vi "Version_4.9_8_on-chip_valves_for25ulSyringe_withModfied_Plunging.vi"() -> ()   [LabVIEW 2020] (continued)
                                n5545 = local read "VISA Refnum in\nfor Pump"() -> (w5935:refnum<visa-resource-name>)
                                n5546 = local read "Volume of Syringe"() -> (w5932:dbl)
                                n5547 = call "GoToAbsolutePosition(SubVI).vi"("Absolute Volume Position in Syringe (in ul)"=0.0, "Volume of Syringe"=w5932, "Resolution of Pumping"=T2."Standard Pumping", "Flow Rate (ul/min)"=150.0, "VISA Refnum in"=w5935) -> ()  [unwired: 6 in, 1 out]
                                }
                                frame #7 {
                                n5548 = local read "Stopper that ends \nthe main loops"() -> (w5936:bool)
                                n5549 = local read "VISA Refnum in\nfor Pump"() -> (w5937:refnum<visa-resource-name>)
                                n5550 = case shown="True" w5936 {
                                frame False {
                                }
                                frame True {
                                n5551 = local read "VISA Refnum in\nfor Pump"() -> (w5938:refnum<visa-resource-name>)
                                n5552 = call "HardStopCurrentProcess (SubVI).vi"("VISA Refnum in"=w5938) -> ()  [unwired: 11 in]
                                }
                                }
                                n5553 = call "ProcessCompletionWaiter (SubVI).vi"("VISA Refnum in"=w5937) -> ()  [unwired: 11 in]
                                }
                                }
                                }
                              }
                            }
                          }
                          frame #21 {
                            n5554 = local read "VISA Refnum in\nfor Pump"() -> (w5940:refnum<visa-resource-name>)
                            n5555 = local read "Port for \nC2-Elution"() -> (w5939:string)
                            n5556 = call "PortChanger (SubVI).vi"("Port Number"=w5939, "VISA Refnum in"=w5940) -> ()  [unwired: 10 in]
                          }
                          frame #22 {
                            n5557 = local read "VISA Refnum in\nfor Pump"() -> (w5941:refnum<visa-resource-name>)
                            n5558 = call "ProcessCompletionWaiter (SubVI).vi"("VISA Refnum in"=w5941) -> ()  [unwired: 11 in]
                          }
                          frame #23 {
                            n5559 = local read "Buffer-C2 PickUp \nFlow Rate (ul/min)"() -> (w5945:dbl)
                            n5560 = local read "Buffer-C2 Pumping\nResolution"() -> (w5944:T2)
                            n5561 = local read "VISA Refnum in\nfor Pump"() -> (w5947:refnum<visa-resource-name>)
                            n5562 = local read "Buffer-C2 Volume \nto be Pumped"() -> (w5943:dbl)
                            n5563 = local read "Volume of Syringe"() -> (w5946:dbl)
                            n5564 = call "RPickUp(SubVI).vi"("Volume to be picked up"=w5943, "Volume of Syringe"=w5946, "Resolution of PickUP"=w5944, "PickUp Flow Rate (ul/min)"=w5945, "VISA Refnum in"=w5947) -> ()  [unwired: 6 in, 1 out]
                            n5565 = local write "SEC On"(TRUE ("SEC On")) -> ()
                          }
                          frame #24 {
                            n5566 = local read "Stopper that ends \nthe main loops"() -> (w5948:bool)
                            n5567 = local read "VISA Refnum in\nfor Pump"() -> (w5949:refnum<visa-resource-name>)
                            n5568 = case shown="True" w5948 {
                              frame False {
                              }
                              frame True {
                                n5569 = local read "VISA Refnum in\nfor Pump"() -> (w5950:refnum<visa-resource-name>)
                                n5570 = call "HardStopCurrentProcess (SubVI).vi"("VISA Refnum in"=w5950) -> ()  [unwired: 11 in]
                              }
                            }
                            n5571 = call "ProcessCompletionWaiter (SubVI).vi"("VISA Refnum in"=w5949) -> ()  [unwired: 11 in]
                          }
                          frame #25 {
                            # "Reads the initial Plunger Position for computing the volume dispensed"
                            n5572 = local read "VISA Refnum in\nfor Pump"() -> (w5952:refnum<visa-resource-name>)
                            n5573 = call "AbsolutePlungerPosition (SubVI).vi"("VISA Refnum in"=w5952) -> ("Plunger Position"=w5951:i32)  [unwired: 10 in]
                            n5574 = local write "Initial Plunger Position"(w5951) -> ()
                          }
                          frame #26 {
                            # "Switch to Port-10"
                            # "Port-10 of the pump is conncted to column-2 of chip"
                            n5575 = local read "VISA Refnum in\nfor Pump"() -> (w5954:refnum<visa-resource-name>)
                            n5576 = call "PortChanger (SubVI).vi"("Port Number"="10", "VISA Refnum in"=w5954) -> ()  [unwired: 10 in]
                          }
                          frame #27 {
                            n5577 = local read "Stopper that ends \nthe main loops"() -> (w5955:bool)
                            n5578 = local read "VISA Refnum in\nfor Pump"() -> (w5956:refnum<visa-resource-name>)
                            n5579 = call "ProcessCompletionWaiter (SubVI).vi"("VISA Refnum in"=w5956) -> ()  [unwired: 11 in]
                            n5580 = case shown="True" w5955 {
                              frame False {
                              }
                              frame True {
                                n5581 = local read "VISA Refnum in\nfor Pump"() -> (w5957:refnum<visa-resource-name>)
                                n5582 = call "HardStopCurrentProcess (SubVI).vi"("VISA Refnum in"=w5957) -> ()  [unwired: 11 in]
                              }
                            }
                          }
                          frame #28 {
                            # "Keeps the AMF valve after column-1 open and valve after column-2 closed"
                            n5583 = local read "Buffer-C2 Dispense\nFlow Rate (ul/min)"() -> (w5970:dbl)
                            n5584 = local read "Buffer-C2 Pumping\nResolution"() -> (w5969:T2)
                            n5585 = local read "VISA Refnum in\nfor Pump"() -> (w5972:refnum<visa-resource-name>)
                            n5586 = local write "Pause Data Collection"(FALSE ("Pause Data Collection")) -> ()
                            n5587 = local read "Volume of Syringe"() -> (w5971:dbl)
                            n5588 = call "GoToAbsolutePosition(SubVI).vi"("Absolute Volume Position in Syringe (in ul)"=0.0 ("Volume to be Dispensed"), "Volume of Syringe"=w5971, "Resolution of Pumping"=w5969, "Flow Rate (ul/min)"=w5970, "VISA Refnum in"=w5972) -> ()  [unwired: 6 in, 1 out]
                            n5589 = local write "Valve V1 Open"(FALSE ("Valve V1 Open")) -> ()
                            n5590 = local write "Valve V2 Open"(TRUE ("Valve V2 Open")) -> ()
                            n5591 = local write "Valve V3 Open"(TRUE ("Valve V3 Open")) -> ()
                            n5592 = local write "Valve V4 Open"(FALSE ("Valve V4 Open")) -> ()
                            n5593 = local write "External Valve \nOpen"(TRUE ("External Valve \nOpen")) -> ()
                            n5594 = local write "Valve V8 Open"(FALSE ("Valve V8 Open")) -> ()
                            n5595 = local write "Valve V5 Open"(FALSE ("Valve V5 Open")) -> ()
                            n5596 = local write "Valve V6 Open"(FALSE ("Valve V6 Open")) -> ()
                            n5597 = local write "Valve V7 Open"(FALSE ("Valve V7 Open")) -> ()
                          }
                          frame #29 {
                            n5598 = local read "Initial Plunger Position"() -> (w5976:dbl)
                            n5599 = local read "Buffer-C2 Pumping\nResolution"() -> (w5975:T2)
                            n5600 = local read "VISA Refnum in\nfor Pump"() -> (w5977:refnum<visa-resource-name>)
                            n5601 = local read "Volume of Syringe"() -> (w5974:dbl)
                            n5602 = while {
                              tunnel: w5976 -> [w5983]
                              tunnel: w5977 -> [w5982]
                              tunnel: w5975 -> [w5981]
                              tunnel: w5974 -> [w5980]
                              stop <- w5978 stop-if-true
                              n5603 = Wait (ms)(milliseconds to wait=u32 100) -> ()  [unwired: 1 out]
                              n5604 = stacked-sequence {
                                tunnel: w5983 -> [w5989 _]
                                tunnel: w5982 -> [w5988 w6015]
                                tunnel: w5981 -> [w5987 _]
                                tunnel: w5980 -> [w5986 _]
                                tunnel: [_ w6011] -> w5978
                                frame #0 {
                                n5605 = call "AbsolutePlungerPosition (SubVI).vi"("VISA Refnum in"=w5988) -> ("Plunger Position"=w5985:i32)  [unwired: 10 in]
                                n5606 = case shown="\"Standard Pumping\", Default" w5987 {
                                tunnel: w5989 -> [w5994 w6003]
                                tunnel: w5985 -> [w5995 w6002]
                                tunnel: [w5993 w6000] -> w5984
                                tunnel: w5986 -> [w5992 w6001]
                                frame "Standard Pumping", Default {
                                n5607 = Subtract(x=w5994, y=w5995) -> (x-y=w5991:dbl)
                                n5608 = Absolute Value(x=w5991) -> (abs(x)=w5990:dbl)
                                n5609 = Multiply(x=w5990, y=w5992) -> (x*y=w5997:dbl)
                                n5610 = Divide(x=w5997, y=3000.0) -> (x/y=w5993:dbl)
                                }
                                frame "High Resolution Pumping" {
                                n5611 = Subtract(x=w6003, y=w6002) -> (x-y=w5999:dbl)
                                n5612 = Absolute Value(x=w5999) -> (abs(x)=w5998:dbl)
                                n5613 = Multiply(x=w5998, y=w6001) -> (x*y=w6005:dbl)
                                n5614 = Divide(x=w6005, y=24000.0) -> (x/y=w6000:dbl)
                                }
                                }
                                n5615 = local write "Volume being Injected \nin this process"(w5984) -> ()
                                }
                                frame #1 {
                                n5616 = local read "Stopper that ends \nthe main loops"() -> (w6012:bool)
                                n5617 = local read "Divert Buffer-C \ninto Column-2"() -> (w6013:bool)
                                n5618 = local read "Volume being Injected \nin this process"() -> (w6010:dbl)
                                n5619 = call "LSPOneStatus (SubVI).vi"("VISA Refnum in"=w6015) -> ("read buffer"=w6017:string)  [unwired: 10 in]
                                n5620 = call <vilib>:"Trim Whitespace.vi"("string"=w6017) -> ("trimmed string"=w6016:string)  [unwired: 1 in]
                                n5621 = Equal?(x=w6016, y="/0`\u0003") -> (x = y?=w6014:bool)
                                n5622 = Or(x=w6013, y=w6012) -> (x .or. y?=w6008:bool)
                                n5623 = Greater Or Equal?(x=w6010, y=2.0) -> (x >= y?=w6007:bool)
                                n5624 = Or(x=w6008, y=w6007) -> (x .or. y?=w6006:bool)
                                n5625 = Or(x=w6014, y=w6006) -> (x .or. y?=w6011:bool)
                                }
                              }
                            }
                            n5626 = local read "Stopper that ends \nthe main loops"() -> (w5973:bool)
                            n5627 = case shown="True" w5973 {
                              frame False {
                              }
                              frame True {
                                n5628 = local read "VISA Refnum in\nfor Pump"() -> (w6019:refnum<visa-resource-name>)
                                n5629 = call "HardStopCurrentProcess (SubVI).vi"("VISA Refnum in"=w6019) -> ()  [unwired: 11 in]
                              }
                            }
                          }
                          frame #30 {
                            # "Keeps the on-chip valves V4, V5 and V7 open"
                            # "Keeps the AMF valve after column-1 closed and valve after column-2 open"
                            n5630 = local write "Divert Buffer-C \ninto Column-2"(FALSE ("Divert Buffer-C \ninto Column-2")) -> ()
                            n5631 = local write "Valve V3 Open"(TRUE ("Valve V3 Open")) -> ()
                            n5632 = local write "Valve V2 Open"(FALSE ("Valve V2 Open")) -> ()
                            n5633 = local write "Valve V1 Open"(FALSE ("Valve V1 Open")) -> ()
                            n5634 = local write "Valve V4 Open"(TRUE ("Valve V4 Open")) -> ()
                            n5635 = local write "External Valve \nOpen"(FALSE ("External Valve \nOpen")) -> ()
                            n5636 = local write "Valve V5 Open"(TRUE ("Valve V5 Open")) -> ()
                            n5637 = local write "Valve V6 Open"(FALSE ("Valve V6 Open")) -> ()
                            n5638 = local write "Valve V8 Open"(FALSE ("Valve V8 Open")) -> ()
                            n5639 = local write "Valve V7 Open"(TRUE ("Valve V7 Open")) -> ()
                          }
                          frame #31 {
                            n5640 = local read "Initial Plunger Position"() -> (w6033:dbl)
                            n5641 = local read "Buffer-C2 Pumping\nResolution"() -> (w6032:T2)
                            n5642 = local read "VISA Refnum in\nfor Pump"() -> (w6034:refnum<visa-resource-name>)
                            n5643 = local read "Volume of Syringe"() -> (w6031:dbl)
                            n5644 = while {
                              tunnel: w6033 -> [w6040]
                              tunnel: w6034 -> [w6039]
                              tunnel: w6032 -> [w6038]
                              tunnel: w6031 -> [w6037]
                              stop <- w6035 stop-if-true
                              n5645 = Wait (ms)(milliseconds to wait=u32 100) -> ()  [unwired: 1 out]
                              n5646 = stacked-sequence {
                                tunnel: w6040 -> [w6046 _]
                                tunnel: w6039 -> [w6045 w6068]
                                tunnel: w6038 -> [w6044 _]
                                tunnel: w6037 -> [w6043 _]
                                tunnel: [_ w6066] -> w6035
                                frame #0 {
                                n5647 = call "AbsolutePlungerPosition (SubVI).vi"("VISA Refnum in"=w6045) -> ("Plunger Position"=w6042:i32)  [unwired: 10 in]
                                n5648 = case shown="\"Standard Pumping\", Default" w6044 {
                                tunnel: w6046 -> [w6051 w6060]
                                tunnel: w6042 -> [w6052 w6059]
                                tunnel: [w6050 w6057] -> w6041
                                tunnel: w6043 -> [w6049 w6058]
                                frame "Standard Pumping", Default {
                                n5649 = Subtract(x=w6051, y=w6052) -> (x-y=w6048:dbl)
                                n5650 = Absolute Value(x=w6048) -> (abs(x)=w6047:dbl)
                                n5651 = Multiply(x=w6047, y=w6049) -> (x*y=w6054:dbl)
                                n5652 = Divide(x=w6054, y=3000.0) -> (x/y=w6050:dbl)
                                }
                                frame "High Resolution Pumping" {
                                n5653 = Subtract(x=w6060, y=w6059) -> (x-y=w6056:dbl)
                                n5654 = Absolute Value(x=w6056) -> (abs(x)=w6055:dbl)
                                n5655 = Multiply(x=w6055, y=w6058) -> (x*y=w6062:dbl)
                                n5656 = Divide(x=w6062, y=24000.0) -> (x/y=w6057:dbl)
                                }
                                }
                                n5657 = local write "Volume being Injected \nin this process"(w6041) -> ()
                                }
                                frame #1 {
                                n5658 = call "LSPOneStatus (SubVI).vi"("VISA Refnum in"=w6068) -> ("read buffer"=w6070:string)  [unwired: 10 in]
                                n5659 = call <vilib>:"Trim Whitespace.vi"("string"=w6070) -> ("trimmed string"=w6069:string)  [unwired: 1 in]
                                n5660 = Equal?(x=w6069, y="/0`\u0003") -> (x = y?=w6067:bool)
                                n5661 = local read "Stopper that ends \nthe main loops"() -> (w6064:bool)
                                n5662 = local read "Divert Sample \nonto Grid"() -> (w6065:bool)
                                n5663 = Or(x=w6065, y=w6064) -> (x .or. y?=w6063:bool)
                                n5664 = Or(x=w6067, y=w6063) -> (x .or. y?=w6066:bool)
                                }
                              }
                            }
                            n5665 = local read "Stopper that ends \nthe main loops"() -> (w6030:bool)
                            n5666 = case shown="True" w6030 {
                              frame False {
                              }
                              frame True {
                                n5667 = local read "VISA Refnum in\nfor Pump"() -> (w6072:refnum<visa-resource-name>)
                                n5668 = call "HardStopCurrentProcess (SubVI).vi"("VISA Refnum in"=w6072) -> ()  [unwired: 11 in]
                              }
                            }
                          }
                          frame #32 {
                            n5669 = local read "Volume being Injected \nin this process"() -> (w6075:dbl)
                            n5670 = local read "VISA Refnum in\nfor Pump"() -> (w6077:refnum<visa-resource-name>)
                            n5671 = call "AbsolutePlungerPosition (SubVI).vi"("VISA Refnum in"=w6077) -> ("Plunger Position"=w6076:i32)  [unwired: 10 in]
                            n5672 = local write "Pause Data Collection"(TRUE) -> ()
                            n5673 = local write "True Volume being \ninjected in this\nprocess"(w6075) -> ()
                            n5674 = local write "Position\nNow"(w6076) -> ()
                            n5675 = Wait (ms)(milliseconds to wait=u32 500) -> ()  [unwired: 1 out]
                          }
                          frame #33 {
                            # "Sample Deposition onto EM-Grid"
                            n5676 = local read "Divert Sample \nonto Grid"() -> (w6078:bool)
                            n5677 = case shown="True" w6078 {
                              frame False {
                              }
                              frame True {
                                n5678 = stacked-sequence {
                                frame #0 {
                                # "Discard the initial volume of fluid that is present in the channel prior to detection"
                                n5679 = local read "Buffer-C2 Pumping\nResolution"() -> (w6091:T2)
                                n5680 = local read "Initial Plunger Position"() -> (w6090:dbl)
                                n5681 = local read "VISA Refnum in\nfor Pump"() -> (w6092:refnum<visa-resource-name>)
                                n5682 = local read "Position\nNow"() -> (w6088:dbl)
                                n5683 = local read "Volume of Syringe"() -> (w6089:dbl)
                                n5684 = local write "Pause Data Collection"(FALSE) -> ()
                                n5685 = while {
                                tunnel: w6092 -> [w6102]
                                tunnel: w6091 -> [w6101]
                                tunnel: w6090 -> [w6097]
                                tunnel: w6089 -> [w6100]
                                tunnel: w6088 -> [w6096]
                                stop <- w6098 stop-if-true
                                n5686 = stacked-sequence {
                                tunnel: w6102 -> [w6108 w6130 w6162]
                                tunnel: w6101 -> [w6107 w6129 _]
                                tunnel: w6097 -> [w6105 _ _]
                                tunnel: w6100 -> [w6104 w6127 _]
                                tunnel: [_ _ w6156] -> w6098
                                tunnel: w6096 -> [_ w6125 _]
                                frame #0 {
                                # "From here on 'True Volume being injected \nin this process' represents the true total \nvolume in this process"
                                n5687 = call "AbsolutePlungerPosition (SubVI).vi"("VISA Refnum in"=w6108) -> ("Plunger Position"=w6106:i32)  [unwired: 10 in]
                                n5688 = case shown="..\"Standard Pumping\"" w6107 {
                                tunnel: w6106 -> [w6116 w6124]
                                tunnel: w6105 -> [w6115 w6123]
                                tunnel: w6104 -> [w6112 w6120]
                                tunnel: [w6109 w6117] -> w6103
                                frame .."Standard Pumping" {
                                n5689 = Subtract(x=w6116, y=w6115) -> (x-y=w6114:dbl)
                                n5690 = Absolute Value(x=w6114) -> (abs(x)=w6113:dbl)
                                n5691 = Multiply(x=w6113, y=w6112) -> (x*y=w6111:dbl)
                                n5692 = Divide(x=w6111, y=3000.0) -> (x/y=w6109:dbl)
                                }
                                frame "High Resolution Pumping".. {
                                n5693 = Subtract(x=w6124, y=w6123) -> (x-y=w6122:dbl)
                                n5694 = Absolute Value(x=w6122) -> (abs(x)=w6121:dbl)
                                n5695 = Multiply(x=w6121, y=w6120) -> (x*y=w6119:dbl)
                                n5696 = Divide(x=w6119, y=24000.0) -> (x/y=w6117:dbl)
                                }
                                }
                                n5697 = local write "True Volume being \ninjected in this\nprocess"(w6103) -> ()
                                }
                                frame #1 {
                                # "From here on 'Volume being injected \nin this process' represents the volume \nin this sub process"
                                n5698 = call "AbsolutePlungerPosition (SubVI).vi"("VISA Refnum in"=w6130) -> ("Plunger Position"=w6128:i32)  [unwired: 10 in]
                                n5699 = case shown="..\"Standard Pumping\"" w6129 {
                                tunnel: w6128 -> [w6138 w6146]
                                tunnel: w6125 -> [w6137 w6145]
                                tunnel: w6127 -> [w6134 w6142]
                                tunnel: [w6131 w6139] -> w6126
                                frame .."Standard Pumping" {
                                n5700 = Subtract(x=w6138, y=w6137) -> (x-y=w6136:dbl)
                                n5701 = Absolute Value(x=w6136) -> (abs(x)=w6135:dbl)
                                n5702 = Multiply(x=w6135, y=w6134) -> (x*y=w6133:dbl)
                                n5703 = Divide(x=w6133, y=3000.0) -> (x/y=w6131:dbl)
                                }
                                frame "High Resolution Pumping".. {
                                n5704 = Subtract(x=w6146, y=w6145) -> (x-y=w6144:dbl)
                                n5705 = Absolute Value(x=w6144) -> (abs(x)=w6143:dbl)
                                n5706 = Multiply(x=w6143, y=w6142) -> (x*y=w6141:dbl)
                                n5707 = Divide(x=w6141, y=24000.0) -> (x/y=w6139:dbl)
                                }
                                }
                                n5708 = local write "Volume being Injected \nin this process"(w6126) -> ()
                                }
                                frame #2 {
                                n5709 = local read "Discard Volume"() -> (w6150:dbl)
                                n5710 = local read "Discard fluid \nprior to 1st \ndeposition"() -> (w6155:bool)
                                n5711 = local read "Volume being Injected \nin this process"() -> (w6154:dbl)
                                n5712 = Greater Or Equal?(x=w6154, y=w6150) -> (x >= y?=w6152:bool)
                                n5713 = call "AbsolutePlungerPositionStatus (SubVI).vi"("VISA Refnum in"=w6162) -> ("read buffer"=w6161:string)  [unwired: 10 in]
                                n5714 = local read "Stop for End of \nExperiment \nand Data Writing"() -> (w6149:bool)
                                n5715 = call <vilib>:"Trim Whitespace.vi"("string"=w6161) -> ("trimmed string"=w6160:string)  [unwired: 1 in]
                                n5716 = Not(x=w6155) -> (.not. x?=w6153:bool)
                                n5717 = Equal?(x=w6160, y="/0`\u0003") -> (x = y?=w6158:bool)
                                n5718 = Or(x=w6153, y=w6152) -> (x .or. y?=w6151:bool)
                                n5719 = local read "Re-SEC"() -> (w6148:bool)
                                n5720 = Or(x=w6149, y=w6148) -> (x .or. y?=w6147:bool)
                                n5721 = Or(x=w6151, y=w6147) -> (x .or. y?=w6157:bool)
                                n5722 = Or(x=w6158, y=w6157) -> (x .or. y?=w6156:bool)
                                }
                                }
                                n5723 = Wait (ms)(milliseconds to wait=u32 100) -> ()  [unwired: 1 out]
                                }
                                n5724 = local write "Valve V4 Open"(TRUE ("Valve V4 Open")) -> ()
                                n5725 = local write "Valve V3 Open"(TRUE ("Valve V3 Open")) -> ()
                                n5726 = local write "Valve V2 Open"(FALSE ("Valve V2 Open")) -> ()
                                n5727 = local write "Valve V1 Open"(FALSE ("Valve V1 Open")) -> ()
                                n5728 = local write "External Valve \nOpen"(FALSE ("External Valve \nOpen")) -> ()
                                n5729 = local write "Valve V5 Open"(TRUE ("Valve V5 Open")) -> ()
                                n5730 = local write "Valve V6 Open"(TRUE ("Valve V6 Open")) -> ()
                                n5731 = local write "Valve V8 Open"(FALSE ("Valve V8 Open")) -> ()
                                n5732 = local write "Valve V7 Open"(FALSE ("Valve V7 Open")) -> ()
                                n5733 = local write "Volume being Injected \nin this process"(0.0) -> ()
                                }
                                frame #1 {
                                # "Keeps the on-chip valve V1, V2 and V3 closed,\nHalts also deposition onto the grid\nand waits for the 1st redeposit command. Once the command is issued\nit starts pumpoing and moves onto the next frame"
                                n5734 = stacked-sequence {
                                frame #0 {
                                n5735 = local write "Valve V5 Open"(FALSE ("Valve V5 Open")) -> ()
                                n5736 = local write "Valve V1 Open"(FALSE ("Valve V1 Open")) -> ()
                                n5737 = local read "VISA Refnum in\nfor Pump"() -> (w6174:refnum<visa-resource-name>)
                                n5738 = local write "Valve V2 Open"(FALSE ("Valve V2 Open")) -> ()
                                n5739 = local write "Valve V6 Open"(FALSE ("Valve V6 Open")) -> ()
                                n5740 = local write "Re-deposit Sample\nonto Grid"(FALSE ("Redeposit Sample\nonto Grid")) -> ()
                                n5741 = local write "Pause Data Collection"(TRUE ("Pause Data Collection")) -> ()
                                n5742 = call "HardStopCurrentProcess (SubVI).vi"("VISA Refnum in"=w6174) -> ()  [unwired: 11 in]
                                n5743 = local write "Valve V7 Open"(FALSE ("Valve V7 Open")) -> ()
                                n5744 = local write "Valve V3 Open"(FALSE ("Valve V3 Open")) -> ()
                                n5745 = local write "External Valve \nOpen"(FALSE ("External Valve \nOpen")) -> ()
                                n5746 = local write "Valve V4 Open"(FALSE ("Valve V4 Open")) -> ()
                                n5747 = local write "Valve V8 Open"(FALSE ("Valve V8 Open")) -> ()
                                }
                                frame #1 {
                                n5748 = while {
                                stop <- w6180 stop-if-true
                                n5749 = local read "Stop for End of \nExperiment \nand Data Writing"() -> (w6178:bool)
                                n5750 = local read "Re-SEC"() -> (w6179:bool)
                                n5751 = local read "Re-deposit Sample\nonto Grid"() -> (w6181:bool)
                                n5752 = Or(x=w6178, y=w6179) -> (x .or. y?=w6177:bool)
                                n5753 = Or(x=w6181, y=w6177) -> (x .or. y?=w6180:bool)
                                }
                                n5754 = local write "Discard fluid \nprior to 1st \ndeposition"(FALSE ("Discard fluid \nprior to 1st \ndeposition")) -> ()
                                n5755 = One Button Dialog(message="Do you want to deposit sample on another grid? If yes, turn on 'Re-deposit Sample onto Grid'. Else turn on Re-SEC to do SEC again or STOP to end the experiment") -> ()  [unwired: 1 in, 1 out]
                                }
                                frame #2 {
                                n5756 = local write "Valve V6 Open"(TRUE ("Valve V3 Open")) -> ()
                                n5757 = local write "Valve V4 Open"(TRUE ("Valve V1 Open")) -> ()
                                n5758 = local write "Valve V5 Open"(TRUE ("Valve V2 Open")) -> ()
                                n5759 = local write "Valve V3 Open"(TRUE ("Valve V3 Open")) -> ()
                                n5760 = local write "Valve V7 Open"(FALSE ("Valve V7 Open")) -> ()
                                }
                                frame #3 {
                                n5761 = local read "Re-deposit Sample\nonto Grid"() -> (w6187:bool)
                                n5762 = case shown="True" w6187 {
                                frame False {
                                n5763 = local write "Suction On/Off"(FALSE ("Suction On/Off")) -> ()
                                }
                                frame True {
                                n5764 = stacked-sequence {
                                frame #0 {
                                n5765 = local read "VISA Refnum in\nfor Pump"() -> (w6190:refnum<visa-resource-name>)
                                n5766 = call "AbsolutePlungerPosition (SubVI).vi"("VISA Refnum in"=w6190) -> ("Plunger Position"=w6189:i32)  [unwired: 10 in]
                                n5767 = local write "Position\nNow"(w6189) -> ()
                                }
                                frame #1 {
                                n5768 = local read "Buffer-C2 Pumping\nResolution"() -> (w6192:T2)
                                n5769 = case shown="\"Standard Pumping\", Default" w6192 {
                                tunnel: [w6193 w6204] -> w6191
                                frame "Standard Pumping", Default {
                                n5770 = local read "Buffer-C2 Volume \nto be Pumped"() -> (w6196:dbl)
                                n5771 = local read "Volume of Syringe"() -> (w6199:dbl)
                                n5772 = local read "Initial Plunger Position"() -> (w6203:dbl)
                                n5773 = local read "Position\nNow"() -> (w6202:dbl)
                                n5774 = Subtract(x=w6203, y=w6202) -> (x-y=w6201:dbl)
                                n5775 = Absolute Value(x=w6201) -> (abs(x)=w6200:dbl)
                                n5776 = Multiply(x=w6200, y=w6199) -> (x*y=w6198:dbl)
                                n5777 = Divide(x=w6198, y=3000.0) -> (x/y=w6195:dbl)
                                n5778 = Subtract(x=w6195, y=w6196) -> (x-y=w6194:dbl)
                                n5779 = Absolute Value(x=w6194) -> (abs(x)=w6193:dbl)
                                }
                                frame "High Resolution Pumping" {
                                n5780 = local read "Buffer-C2 Volume \nto be Pumped"() -> (w6207:dbl)
                                n5781 = local read "Volume of Syringe"() -> (w6210:dbl)
                                n5782 = local read "Initial Plunger Position"() -> (w6214:dbl)
                                n5783 = local read "Position\nNow"() -> (w6213:dbl)
                                n5784 = Subtract(x=w6214, y=w6213) -> (x-y=w6212:dbl)
                                n5785 = Absolute Value(x=w6212) -> (abs(x)=w6211:dbl)
                                n5786 = Multiply(x=w6211, y=w6210) -> (x*y=w6209:dbl)
                                n5787 = Divide(x=w6209, y=24000.0) -> (x/y=w6206:dbl)
                                n5788 = Subtract(x=w6206, y=w6207) -> (x-y=w6205:dbl)
                                n5789 = Absolute Value(x=w6205) -> (abs(x)=w6204:dbl)
                                }
                                }
                                n5790 = local write "Buffer-C Volume\nleft to be Pumped"(w6191) -> ()
                                }
                                frame #2 {
                                n5791 = local read "Buffer-C2 Dispense\nFlow Rate (ul/min)"() -> (w6218:dbl)
                                n5792 = local read "Buffer-C2 Pumping\nResolution"() -> (w6217:T2)
                                n5793 = local read "VISA Refnum in\nfor Pump"() -> (w6220:refnum<visa-resource-name>)
                                n5794 = local read "Volume of Syringe"() -> (w6219:dbl)
                                n5795 = call "GoToAbsolutePosition(SubVI).vi"("Absolute Volume Position in Syringe (in ul)"=0.0, "Volume of Syringe"=w6219, "Resolution of Pumping"=w6217, "Flow Rate (ul/min)"=w6218, "VISA Refnum in"=w6220) -> ()  [unwired: 6 in, 1 out]
                                n5796 = local write "Suction On/Off"(FALSE ("Suction On/Off")) -> ()
                                }
                                }
                                }
                                }
                                }
                                frame #4 {
                                n5797 = local read "Stop for End of \nExperiment \nand Data Writing"() -> (w6223:bool)
                                n5798 = local read "Re-SEC"() -> (w6222:bool)
                                n5799 = Or(x=w6223, y=w6222) -> (x .or. y?=w6221:bool)
                                n5800 = case shown="True" w6221 {
                                frame False {
                                }
                                frame True {
                                n5801 = local read "VISA Refnum in\nfor Pump"() -> (w6224:refnum<visa-resource-name>)
                                n5802 = call "HardStopCurrentProcess (SubVI).vi"("VISA Refnum in"=w6224) -> ()  [unwired: 11 in]
                                }
                                }
                                }
                                }
                                }
                                frame #2 {
                                # "Keeps the on-chip valve V1, V2 Open and V3 closed"
                                n5803 = while {
                                stop <- w6230 stop-if-true
                                n5804 = local read "Suction On/Off"() -> (w6231:bool)
                                n5805 = case shown="True" w6231 {
                                frame False {
                                n5806 = local read "Buffer-C2 Pumping\nResolution"() -> (w6237:T2)
                                n5807 = local read "Initial Plunger Position"() -> (w6236:dbl)
                                n5808 = local read "VISA Refnum in\nfor Pump"() -> (w6238:refnum<visa-resource-name>)
                                n5809 = local read "Position\nNow"() -> (w6234:dbl)
                                n5810 = local read "Volume of Syringe"() -> (w6235:dbl)
                                n5811 = local write "Volume being Injected \nin this process"(0.0) -> ()
                                n5812 = local write "Pause Data Collection"(FALSE) -> ()
                                n5813 = while {
                                tunnel: w6238 -> [w6245]
                                tunnel: w6237 -> [w6244]
                                tunnel: w6236 -> [w6240]
                                tunnel: w6235 -> [w6243]
                                tunnel: w6234 -> [w6239]
                                stop <- w6241 stop-if-true
                                n5814 = stacked-sequence {
                                tunnel: w6245 -> [w6251 w6273 w6300]
                                tunnel: w6244 -> [w6250 w6272 _]
                                tunnel: w6240 -> [w6248 _ _]
                                tunnel: w6243 -> [w6247 w6270 _]
                                tunnel: [_ _ w6293] -> w6241
                                tunnel: w6239 -> [_ w6268 _]
                                frame #0 {
                                # "From here on 'True Volume being injected \nin this process' represents the true total \nvolume in this process"
                                n5815 = call "AbsolutePlungerPosition (SubVI).vi"("VISA Refnum in"=w6251) -> ("Plunger Position"=w6249:i32)  [unwired: 10 in]
                                n5816 = case shown="..\"Standard Pumping\"" w6250 {
                                tunnel: w6249 -> [w6259 w6267]
                                tunnel: w6248 -> [w6258 w6266]
                                tunnel: w6247 -> [w6255 w6263]
                                tunnel: [w6252 w6260] -> w6246
                                frame .."Standard Pumping" {
                                n5817 = Subtract(x=w6259, y=w6258) -> (x-y=w6257:dbl)
                                n5818 = Absolute Value(x=w6257) -> (abs(x)=w6256:dbl)
                                n5819 = Multiply(x=w6256, y=w6255) -> (x*y=w6254:dbl)
                                n5820 = Divide(x=w6254, y=3000.0) -> (x/y=w6252:dbl)
                                }
                                frame "High Resolution Pumping".. {
                                n5821 = Subtract(x=w6267, y=w6266) -> (x-y=w6265:dbl)
                                n5822 = Absolute Value(x=w6265) -> (abs(x)=w6264:dbl)
                                n5823 = Multiply(x=w6264, y=w6263) -> (x*y=w6262:dbl)
                                n5824 = Divide(x=w6262, y=24000.0) -> (x/y=w6260:dbl)
                                }
                                }
                                n5825 = local write "True Volume being \ninjected in this\nprocess"(w6246) -> ()
                                }
                                frame #1 {
                                # "From here on 'Volume being injected \nin this process' represents the volume \nin this sub process"
                                n5826 = call "AbsolutePlungerPosition (SubVI).vi"("VISA Refnum in"=w6273) -> ("Plunger Position"=w6271:i32)  [unwired: 10 in]
                                n5827 = case shown="\"High Resolution Pumping\".." w6272 {
                                tunnel: w6271 -> [w6281 w6289]
                                tunnel: w6268 -> [w6280 w6288]
                                tunnel: w6270 -> [w6277 w6285]
                                tunnel: [w6274 w6282] -> w6269
                                frame .."Standard Pumping" {
                                n5828 = Subtract(x=w6281, y=w6280) -> (x-y=w6279:dbl)
                                n5829 = Absolute Value(x=w6279) -> (abs(x)=w6278:dbl)
                                n5830 = Multiply(x=w6278, y=w6277) -> (x*y=w6276:dbl)
                                n5831 = Divide(x=w6276, y=3000.0) -> (x/y=w6274:dbl)
                                }
                                frame "High Resolution Pumping".. {
                                n5832 = Subtract(x=w6289, y=w6288) -> (x-y=w6287:dbl)
                                n5833 = Absolute Value(x=w6287) -> (abs(x)=w6286:dbl)
                                n5834 = Multiply(x=w6286, y=w6285) -> (x*y=w6284:dbl)
                                n5835 = Divide(x=w6284, y=24000.0) -> (x/y=w6282:dbl)
                                }
                                }
                                n5836 = local write "Volume being Injected \nin this process"(w6269) -> ()
                                }
                                frame #2 {
                                n5837 = local read "Stop for End of \nExperiment \nand Data Writing"() -> (w6292:bool)
                                n5838 = local read "Re-SEC"() -> (w6291:bool)
                                n5839 = local read "Suction On/Off"() -> (w6296:bool)
                                n5840 = call "AbsolutePlungerPositionStatus (SubVI).vi"("VISA Refnum in"=w6300) -> ("read buffer"=w6299:string)  [unwired: 10 in]
                                n5841 = call <vilib>:"Trim Whitespace.vi"("string"=w6299) -> ("trimmed string"=w6298:string)  [unwired: 1 in]
                                n5842 = Equal?(x=w6298, y="/0`\u0003") -> (x = y?=w6295:bool)
                                n5843 = Or(x=w6292, y=w6291) -> (x .or. y?=w6290:bool)
                                n5844 = Or(x=w6296, y=w6290) -> (x .or. y?=w6294:bool)
                                n5845 = Or(x=w6295, y=w6294) -> (x .or. y?=w6293:bool)
                                }
                                }
                                n5846 = Wait (ms)(milliseconds to wait=u32 100) -> ()  [unwired: 1 out]
                                }
                                }
                                frame True {
                                n5847 = stacked-sequence {
                                frame #0 {
                                n5848 = local write "Valve V3 Open"(FALSE ("Valve V3 Open")) -> ()
                                n5849 = local read "Suction Pressure\nfor EM-grid \nDeposition (mbar)"() -> (w6307:sgl)
                                n5850 = local write "Valve V4 Open"(FALSE ("Valve V4 Open")) -> ()
                                n5851 = local read "VISA Refnum in\nfor Pump"() -> (w6310:refnum<visa-resource-name>)
                                n5852 = local write "Valve V5 Open"(FALSE ("Valve V1 Open")) -> ()
                                n5853 = local write "Suction pressure \nfor grid deposition"(w6307) -> ()
                                n5854 = local write "Re-deposit Sample\nonto Grid"(FALSE ("Redeposit Sample\nonto Grid")) -> ()
                                n5855 = local write "Pause Data Collection"(TRUE ("Pause Data Collection")) -> ()
                                n5856 = call "HardStopCurrentProcess (SubVI).vi"("VISA Refnum in"=w6310) -> ()  [unwired: 11 in]
                                n5857 = local write "Valve V6 Open"(TRUE ("Valve V2 Open")) -> ()
                                n5858 = local write "Valve V7 Open"(TRUE ("Valve V3 Open")) -> ()
                                n5859 = local write "External Valve \nOpen"(FALSE ("External Valve \nOpen")) -> ()
                                }
                                frame #1 {
                                n5860 = while {
                                stop <- w6313 stop-if-true
                                n5861 = local read "Stop for End of \nExperiment \nand Data Writing"() -> (w6314:bool)
                                n5862 = local read "Suction Pressure\nfor EM-grid \nDeposition (mbar)"() -> (w6311:sgl)
                                n5863 = call <vilib>:"fgt set pressure.vi"("pressure"=w6311, "pressureIndex"=u32 1) -> ()  [unwired: 9 in, 1 out]
                                n5864 = local read "Suction On/Off"() -> (w6316:bool)
                                n5865 = Not(x=w6316) -> (.not. x?=w6315:bool)
                                n5866 = Wait (ms)(milliseconds to wait=u32 100) -> ()  [unwired: 1 out]
                                n5867 = Or(x=w6315, y=w6314) -> (x .or. y?=w6313:bool)
                                }
                                }
                                frame #2 {
                                n5868 = for {
                                N: 2 -> [_]
                                n5869 = while {
                                stop <- w6326 stop-if-true
                                n5870 = local read "Stop for End of \nExperiment \nand Data Writing"() -> (w6322:bool)
                                n5871 = local read "Suction On/Off"() -> (w6324:bool)
                                n5872 = call <vilib>:"fgt set pressure.vi"("pressure"=sgl 0.0, "pressureIndex"=u32 1) -> ()  [unwired: 9 in, 1 out]
                                n5873 = Not(x=w6324) -> (.not. x?=w6323:bool)
                                n5874 = Wait (ms)(milliseconds to wait=u32 100) -> ()  [unwired: 1 out]
                                n5875 = Or(x=w6323, y=w6322) -> (x .or. y?=w6326:bool)
                                }
                                n5876 = Wait (ms)(milliseconds to wait=u32 400) -> ()  [unwired: 1 out]
                                }
                                }
                                frame #3 {
                                n5877 = local read "Automatic purging \nof capillary after \ngrid deposition"() -> (w6327:bool)
                                n5878 = case shown="True" w6327 {
                                frame False {
                                }
                                frame True {
                                n5879 = stacked-sequence {
                                frame #0 {
                                n5880 = local read "VISA Refnum in\nfor Pump"() -> (w6329:refnum<visa-resource-name>)
                                n5881 = call "AbsolutePlungerPosition (SubVI).vi"("VISA Refnum in"=w6329) -> ("Plunger Position"=w6328:i32)  [unwired: 10 in]
                                n5882 = local write "Position\nNow"(w6328) -> ()
                                }
                                frame #1 {
                                n5883 = local read "Buffer-C2 Pumping\nResolution"() -> (w6331:T2)
                                n5884 = case shown="\"Standard Pumping\", Default" w6331 {
                                tunnel: [w6332 w6343] -> w6330
                                frame "Standard Pumping", Default {
                                n5885 = local read "Buffer-C2 Volume \nto be Pumped"() -> (w6335:dbl)
                                n5886 = local read "Volume of Syringe"() -> (w6338:dbl)
                                n5887 = local read "Initial Plunger Position"() -> (w6342:dbl)
                                n5888 = local read "Position\nNow"() -> (w6341:dbl)
                                n5889 = Subtract(x=w6342, y=w6341) -> (x-y=w6340:dbl)
                                n5890 = Absolute Value(x=w6340) -> (abs(x)=w6339:dbl)
                                n5891 = Multiply(x=w6339, y=w6338) -> (x*y=w6337:dbl)
                                n5892 = Divide(x=w6337, y=3000.0) -> (x/y=w6334:dbl)
                                n5893 = Subtract(x=w6334, y=w6335) -> (x-y=w6333:dbl)
                                n5894 = Absolute Value(x=w6333) -> (abs(x)=w6332:dbl)
                                }
                                frame "High Resolution Pumping" {
                                n5895 = local read "Buffer-C2 Volume \nto be Pumped"() -> (w6346:dbl)
                                n5896 = local read "Volume of Syringe"() -> (w6349:dbl)
                                n5897 = local read "Initial Plunger Position"() -> (w6353:dbl)
                                n5898 = local read "Position\nNow"() -> (w6352:dbl)
                                n5899 = Subtract(x=w6353, y=w6352) -> (x-y=w6351:dbl)
                                n5900 = Absolute Value(x=w6351) -> (abs(x)=w6350:dbl)
                                n5901 = Multiply(x=w6350, y=w6349) -> (x*y=w6348:dbl)
                                n5902 = Divide(x=w6348, y=24000.0) -> (x/y=w6345:dbl)
                                n5903 = Subtract(x=w6345, y=w6346) -> (x-y=w6344:dbl)
                                n5904 = Absolute Value(x=w6344) -> (abs(x)=w6343:dbl)
                                }
                                }
                                n5905 = local write "Buffer-C Volume\nleft to be Pumped"(w6330) -> ()
                                }
                                frame #2 {
                                n5906 = local read "Buffer-C2 Dispense\nFlow Rate (ul/min)"() -> (w6362:dbl)
                                n5907 = local read "Buffer-C2 Pumping\nResolution"() -> (w6361:T2)
                                n5908 = local read "VISA Refnum in\nfor Pump"() -> (w6364:refnum<visa-resource-name>)
                                n5909 = local read "Volume of Syringe"() -> (w6363:dbl)
                                n5910 = call "GoToAbsolutePosition(SubVI).vi"("Absolute Volume Position in Syringe (in ul)"=0.0, "Volume of Syringe"=w6363, "Resolution of Pumping"=w6361, "Flow Rate (ul/min)"=w6362, "VISA Refnum in"=w6364) -> ()  [unwired: 6 in, 1 out]
                                n5911 = local write "External Valve \nOpen"(FALSE ("External Valve \nOpen")) -> ()
                                n5912 = local write "Valve V3 Open"(TRUE ("Valve V3 Open")) -> ()
                                n5913 = local write "Valve V7 Open"(FALSE ("Valve V3 Open")) -> ()
                                n5914 = local write "Valve V5 Open"(TRUE ("Valve V1 Open")) -> ()
                                n5915 = local write "Valve V6 Open"(TRUE ("Valve V2 Open")) -> ()
                                n5916 = local write "Valve V4 Open"(TRUE ("Valve V4 Open")) -> ()
                                }
                                frame #3 {
                                n5917 = local read "Buffer-C2 Pumping\nResolution"() -> (w6370:T2)
                                n5918 = local read "Initial Plunger Position"() -> (w6369:dbl)
                                n5919 = local read "VISA Refnum in\nfor Pump"() -> (w6371:refnum<visa-resource-name>)
                                n5920 = local read "Position\nNow"() -> (w6367:dbl)
                                n5921 = local read "Volume of Syringe"() -> (w6368:dbl)
                                n5922 = local write "Volume being Injected \nin this process"(0.0) -> ()
                                n5923 = local write "Pause Data Collection"(FALSE) -> ()
                                n5924 = while {
                                tunnel: w6371 -> [w6378]
                                tunnel: w6370 -> [w6377]
                                tunnel: w6369 -> [w6373]
                                tunnel: w6368 -> [w6376]
                                tunnel: w6367 -> [w6372]
                                stop <- w6374 stop-if-true
                                n5925 = stacked-sequence {
                                tunnel: w6378 -> [w6384 w6406 w6435]
                                tunnel: w6377 -> [w6383 w6405 _]
                                tunnel: w6373 -> [w6381 _ _]
                                tunnel: w6376 -> [w6380 w6403 _]
                                tunnel: [_ _ w6429] -> w6374
                                tunnel: w6372 -> [_ w6401 _]
                                frame #0 {
                                # "From here on 'True Volume being injected \nin this process' represents the true total \nvolume in this process"
                                n5926 = call "AbsolutePlungerPosition (SubVI).vi"("VISA Refnum in"=w6384) -> ("Plunger Position"=w6382:i32)  [unwired: 10 in]
                                n5927 = case shown="..\"Standard Pumping\"" w6383 {
                                tunnel: w6382 -> [w6392 w6400]
                                tunnel: w6381 -> [w6391 w6399]
                                tunnel: w6380 -> [w6388 w6396]
                                tunnel: [w6385 w6393] -> w6379
                                frame .."Standard Pumping" {
                                n5928 = Subtract(x=w6392, y=w6391) -> (x-y=w6390:dbl)
                                n5929 = Absolute Value(x=w6390) -> (abs(x)=w6389:dbl)
                                n5930 = Multiply(x=w6389, y=w6388) -> (x*y=w6387:dbl)
                                n5931 = Divide(x=w6387, y=3000.0) -> (x/y=w6385:dbl)
                                }
                                frame "High Resolution Pumping".. {
                                n5932 = Subtract(x=w6400, y=w6399) -> (x-y=w6398:dbl)
                                n5933 = Absolute Value(x=w6398) -> (abs(x)=w6397:dbl)
                                n5934 = Multiply(x=w6397, y=w6396) -> (x*y=w6395:dbl)
                                n5935 = Divide(x=w6395, y=24000.0) -> (x/y=w6393:dbl)
                                }
                                }
                                n5936 = local write "True Volume being \ninjected in this\nprocess"(w6379) -> ()
                                }
                                frame #1 {
                                # "From here on 'Volume being injected \nin this process' represents the volume \nin this sub process"
                                n5937 = call "AbsolutePlungerPosition (SubVI).vi"("VISA Refnum in"=w6406) -> ("Plunger Position"=w6404:i32)  [unwired: 10 in]
                                n5938 = case shown="\"High Resolution Pumping\".." w6405 {
                                tunnel: w6404 -> [w6414 w6422]
                                tunnel: w6401 -> [w6413 w6421]
                                tunnel: w6403 -> [w6410 w6418]
                                tunnel: [w6407 w6415] -> w6402
                                frame .."Standard Pumping" {
                                n5939 = Subtract(x=w6414, y=w6413) -> (x-y=w6412:dbl)
                                n5940 = Absolute Value(x=w6412) -> (abs(x)=w6411:dbl)
                                n5941 = Multiply(x=w6411, y=w6410) -> (x*y=w6409:dbl)
                                n5942 = Divide(x=w6409, y=3000.0) -> (x/y=w6407:dbl)
                                }
                                frame "High Resolution Pumping".. {
                                n5943 = Subtract(x=w6422, y=w6421) -> (x-y=w6420:dbl)
                                n5944 = Absolute Value(x=w6420) -> (abs(x)=w6419:dbl)
                                n5945 = Multiply(x=w6419, y=w6418) -> (x*y=w6417:dbl)
                                n5946 = Divide(x=w6417, y=24000.0) -> (x/y=w6415:dbl)
                                }
                                }
                                n5947 = local write "Volume being Injected \nin this process"(w6402) -> ()
                                }
                                frame #2 {
                                n5948 = local read "Capillary purge \nvolume after every\ngrid plunging"() -> (w6424:dbl)
                                n5949 = local read "Stop for End of \nExperiment \nand Data Writing"() -> (w6428:bool)
                                n5950 = local read "Volume being Injected \nin this process"() -> (w6425:dbl)
                                n5951 = local read "Re-SEC"() -> (w6427:bool)
                                n5952 = call "AbsolutePlungerPositionStatus (SubVI).vi"("VISA Refnum in"=w6435) -> ("read buffer"=w6434:string)  [unwired: 10 in]
                                n5953 = call <vilib>:"Trim Whitespace.vi"("string"=w6434) -> ("trimmed string"=w6433:string)  [unwired: 1 in]
                                n5954 = Greater Or Equal?(x=w6425, y=w6424) -> (x >= y?=w6423:bool)
                                n5955 = Equal?(x=w6433, y="/0`\u0003") -> (x = y?=w6431:bool)
                                n5956 = Or(x=w6428, y=w6427) -> (x .or. y?=w6426:bool)
                                n5957 = Or(x=w6423, y=w6426) -> (x .or. y?=w6430:bool)
                                n5958 = Or(x=w6431, y=w6430) -> (x .or. y?=w6429:bool)
                                }
                                }
                                n5959 = Wait (ms)(milliseconds to wait=u32 100) -> ()  [unwired: 1 out]
                                }
                                }
                                frame #4 {
                                n5960 = local read "VISA Refnum in\nfor Pump"() -> (w6436:refnum<visa-resource-name>)
                                n5961 = call "HardStopCurrentProcess (SubVI).vi"("VISA Refnum in"=w6436) -> ()  [unwired: 11 in]
                                }
                                }
                                }
                                }
                                }
                                frame #4 {
                                n5962 = local write "Valve V3 Open"(FALSE ("Valve V3 Open")) -> ()
                                n5963 = local write "Valve V7 Open"(FALSE ("Valve V3 Open")) -> ()
                                n5964 = local write "Valve V5 Open"(FALSE ("Valve V1 Open")) -> ()
                                n5965 = local write "Valve V6 Open"(FALSE ("Valve V2 Open")) -> ()
                                n5966 = local write "Valve V4 Open"(FALSE ("Valve V4 Open")) -> ()
                                }
                                frame #5 {
                                n5967 = while {
                                stop <- w6446 stop-if-true
                                n5968 = local read "Stop for End of \nExperiment \nand Data Writing"() -> (w6444:bool)
                                n5969 = local read "Re-deposit Sample\nonto Grid"() -> (w6447:bool)
                                n5970 = local read "Re-SEC"() -> (w6445:bool)
                                n5971 = Or(x=w6444, y=w6445) -> (x .or. y?=w6443:bool)
                                n5972 = Or(x=w6447, y=w6443) -> (x .or. y?=w6446:bool)
                                }
                                n5973 = One Button Dialog(message="Do you want to deposit sample on another grid? If yes, turn on 'Re-deposit Sample onto Grid'. Else turn on Re-SEC to do SEC again or STOP to end the experiment") -> ()  [unwired: 1 in, 1 out]
                                }
                                frame #6 {
                                n5974 = local write "Valve V4 Open"(TRUE ("Valve V4 Open")) -> ()
                                n5975 = local write "Valve V3 Open"(TRUE ("Valve V3 Open")) -> ()
                                n5976 = local write "Valve V7 Open"(FALSE ("Valve V3 Open")) -> ()
                                n5977 = local write "Valve V5 Open"(TRUE ("Valve V1 Open")) -> ()
                                n5978 = local write "Valve V6 Open"(TRUE ("Valve V2 Open")) -> ()
                                }
                                frame #7 {
                                n5979 = local read "Re-deposit Sample\nonto Grid"() -> (w6453:bool)
                                n5980 = case shown="True" w6453 {
                                frame False {
                                n5981 = local write "Suction On/Off"(FALSE ("Suction On/Off")) -> ()
                                }
                                frame True {
                                n5982 = stacked-sequence {
                                frame #0 {
                                n5983 = local read "VISA Refnum in\nfor Pump"() -> (w6456:refnum<visa-resource-name>)
                                n5984 = call "AbsolutePlungerPosition (SubVI).vi"("VISA Refnum in"=w6456) -> ("Plunger Position"=w6455:i32)  [unwired: 10 in]
                                n5985 = local write "Position\nNow"(w6455) -> ()
                                }
                                frame #1 {
                                n5986 = local read "Buffer-C2 Pumping\nResolution"() -> (w6458:T2)
                                n5987 = case shown="\"Standard Pumping\", Default" w6458 {
                                tunnel: [w6459 w6470] -> w6457
                                frame "Standard Pumping", Default {
                                n5988 = local read "Buffer-C2 Volume \nto be Pumped"() -> (w6462:dbl)
                                n5989 = local read "Volume of Syringe"() -> (w6465:dbl)
                                n5990 = local read "Initial Plunger Position"() -> (w6469:dbl)
                                n5991 = local read "Position\nNow"() -> (w6468:dbl)
                                n5992 = Subtract(x=w6469, y=w6468) -> (x-y=w6467:dbl)
                                n5993 = Absolute Value(x=w6467) -> (abs(x)=w6466:dbl)
                                n5994 = Multiply(x=w6466, y=w6465) -> (x*y=w6464:dbl)
                                n5995 = Divide(x=w6464, y=3000.0) -> (x/y=w6461:dbl)
                                n5996 = Subtract(x=w6461, y=w6462) -> (x-y=w6460:dbl)
                                n5997 = Absolute Value(x=w6460) -> (abs(x)=w6459:dbl)
                                }
                                frame "High Resolution Pumping" {
                                n5998 = local read "Buffer-C2 Volume \nto be Pumped"() -> (w6473:dbl)
                                n5999 = local read "Volume of Syringe"() -> (w6476:dbl)
                                n6000 = local read "Initial Plunger Position"() -> (w6480:dbl)
                                n6001 = local read "Position\nNow"() -> (w6479:dbl)
                                n6002 = Subtract(x=w6480, y=w6479) -> (x-y=w6478:dbl)
                                n6003 = Absolute Value(x=w6478) -> (abs(x)=w6477:dbl)
                                n6004 = Multiply(x=w6477, y=w6476) -> (x*y=w6475:dbl)
                                n6005 = Divide(x=w6475, y=24000.0) -> (x/y=w6472:dbl)
                                n6006 = Subtract(x=w6472, y=w6473) -> (x-y=w6471:dbl)
                                n6007 = Absolute Value(x=w6471) -> (abs(x)=w6470:dbl)
                                }
                                }
                                n6008 = local write "Buffer-C Volume\nleft to be Pumped"(w6457) -> ()
                                }
                                frame #2 {
                                n6009 = local read "Buffer-C2 Dispense\nFlow Rate (ul/min)"() -> (w6484:dbl)
                                n6010 = local read "Buffer-C2 Pumping\nResolution"() -> (w6483:T2)
                                n6011 = local read "VISA Refnum in\nfor Pump"() -> (w6486:refnum<visa-resource-name>)
                                n6012 = local read "Volume of Syringe"() -> (w6485:dbl)
                                n6013 = call "GoToAbsolutePosition(SubVI).vi"("Absolute Volume Position in Syringe (in ul)"=0.0, "Volume of Syringe"=w6485, "Resolution of Pumping"=w6483, "Flow Rate (ul/min)"=w6484, "VISA Refnum in"=w6486) -> ()  [unwired: 6 in, 1 out]
                                n6014 = local write "Suction On/Off"(FALSE ("Suction On/Off")) -> ()
                                }
                                }
                                }
                                }
                                }
                                frame #8 {
                                n6015 = local read "Stop for End of \nExperiment \nand Data Writing"() -> (w6488:bool)
                                n6016 = local read "Re-SEC"() -> (w6489:bool)
                                n6017 = Or(x=w6488, y=w6489) -> (x .or. y?=w6487:bool)
                                n6018 = case shown="True" w6487 {
                                frame False {
                                }
                                frame True {
                                n6019 = local read "VISA Refnum in\nfor Pump"() -> (w6490:refnum<visa-resource-name>)
                                n6020 = call "HardStopCurrentProcess (SubVI).vi"("VISA Refnum in"=w6490) -> ()  [unwired: 11 in]
                                }
                                }
                                }
                                }
                                }
                                }
                                n6021 = local read "Stop for End of \nExperiment \nand Data Writing"() -> (w6226:bool)
                                n6022 = local read "Divert Sample \nonto Grid"() -> (w6229:bool)
                                n6023 = local read "Re-SEC"() -> (w6227:bool)
                                n6024 = Not(x=w6229) -> (.not. x?=w6228:bool)
                                n6025 = Or(x=w6226, y=w6227) -> (x .or. y?=w6225:bool)
                                n6026 = Or(x=w6228, y=w6225) -> (x .or. y?=w6230:bool)
                                }
                                }
                                }
                                n6027 = local write "Discard fluid \nprior to 1st \ndeposition"(TRUE ("Discard fluid \nprior to 1st \ndeposition")) -> ()
                              }
                            }
                          }
                          frame #34 {
                            n6028 = local read "Stopper that ends \nthe main loops"() -> (w6492:bool)
                            n6029 = local read "Re-SEC"() -> (w6493:bool)
                            n6030 = Wait (ms)(milliseconds to wait=u32 500) -> ()  [unwired: 1 out]
                            n6031 = Or(x=w6492, y=w6493) -> (x .or. y?=w6491:bool)
                            n6032 = case shown="True" w6491 {
                              frame False {
                              }
                              frame True {
                                n6033 = local read "VISA Refnum in\nfor Pump"() -> (w6498:refnum<visa-resource-name>)
                                n6034 = call "HardStopCurrentProcess (SubVI).vi"("VISA Refnum in"=w6498) -> ()  [unwired: 11 in]
                              }
                            }
                            n6035 = local write "Divert Sample \nonto Grid"(FALSE ("Divert Sample \nonto Grid")) -> ()
                            n6036 = local write "Pause Data Collection"(TRUE ("Pause Data Collection")) -> ()
                            n6037 = local write "Start the Process"(FALSE ("Start the Process")) -> ()
                          }
                          frame #35 {
                            n6038 = local read "Stop for End of \nExperiment \nand Data Writing"() -> (w6505:bool)
                            n6039 = local read "Start the Process"() -> (w6504:bool)
                            n6040 = Or(x=w6504, y=w6505) -> (x .or. y?=w6503:bool)
                            n6041 = case shown="False" w6503 {
                              frame False {
                                n6042 = while {
                                stop <- w6511 stop-if-true
                                n6043 = local read "Stop for End of \nExperiment \nand Data Writing"() -> (w6513:bool)
                                n6044 = local read "Start the Process"() -> (w6512:bool)
                                n6045 = Or(x=w6512, y=w6513) -> (x .or. y?=w6511:bool)
                                n6046 = Wait (ms)(milliseconds to wait=u32 100) -> ()  [unwired: 1 out]
                                }
                                n6047 = One Button Dialog(message="Do you want to re-introduce sample into column-2 and elute? If yes, adjust the re-introduction volume into column-2 and elution parameters for column-2 and turn on the 'Start the Process' button . If no, turn on the 'Stop for End of Experiment and Data Writing'.") -> ()  [unwired: 1 in, 1 out]
                              }
                              frame True {
                                n6048 = local read "Stop for End of \nExperiment \nand Data Writing"() -> (w6514:bool)
                                n6049 = case shown="True" w6514 {
                                frame False {
                                }
                                frame True {
                                n6050 = local write "Valve V1 Open"(FALSE ("Valve V1 Open")) -> ()
                                n6051 = local write "Valve V2 Open"(FALSE ("Valve V2 Open")) -> ()
                                n6052 = local write "Valve V4 Open"(FALSE ("Valve V4 Open")) -> ()
                                n6053 = local write "Valve V3 Open"(FALSE ("Valve V3 Open")) -> ()
                                n6054 = local write "Valve V5 Open"(FALSE ("Valve V5 Open")) -> ()
                                n6055 = local write "Valve V6 Open"(FALSE ("Valve V6 Open")) -> ()
                                n6056 = local write "Valve V7 Open"(FALSE ("Valve V7 Open")) -> ()
                                }
                                }
                              }
                            }
                            n6057 = local write "Sample Volume Diverted\ninto Column-2"(0.0 ("Sample Volume Diverted\ninto Column-2")) -> ()
                            n6058 = local write "Buffer-C Volume\nleft to be Pumped"(0.0 ("Buffer-C Volume\nleft to be Pumped")) -> ()
                            n6059 = local write "Vol_previous"(0.0 ("Vol_previous")) -> ()
                            n6060 = local write "Vol_now"(0.0 ("Vol_now")) -> ()
                            n6061 = local write "Elution of Column-2"(FALSE ("Elution of Column-2")) -> ()
                            n6062 = local write "SEC On"(FALSE ("SEC On")) -> ()
